vi "Configure TLS.vi"(4 "Cert Chain Format":enum32{"X.509 (PEM)"}(ring), 6 "Cert Chain Path":path, 7 "Private Key Password":string, 8 "error in (no error)":errorcluster, 9 "Private Key Format":enum32{"PKCS#8 (PEM)", "PKCS#8 (DER)"}(ring), 10 "Private Key Path":path, 11 "Websocket Server in":refnum<class "Websocket Server.lvclass">) -> (0 "error out":errorcluster, 3 "Websocket Server out":refnum<class "Websocket Server.lvclass">)   [LabVIEW 2020, in "Stream-Websocket.lvlib" / "Websocket Server.lvclass"]
uses:
  Websocket Server.lvclass
  Websocket Server.lvclass/Websocket Server.ctl
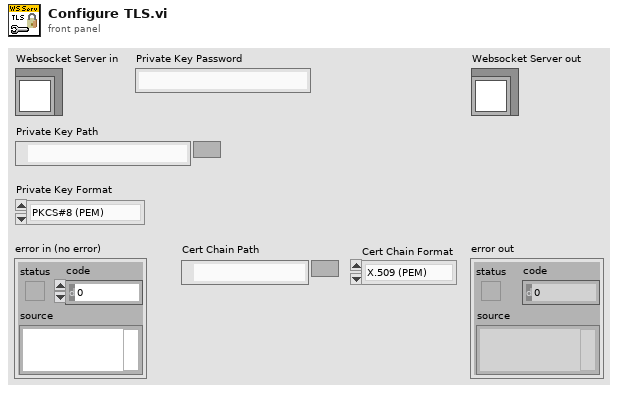
[diagram p1: front panel]
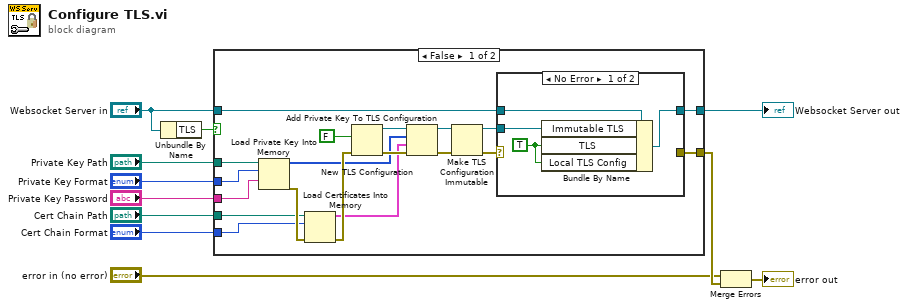
[diagram p0: block diagram]
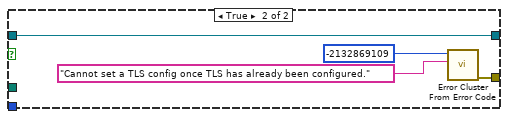
[diagram p3: hidden frame]
diagram:
  n1 = Unbundle By Name("Websocket Server in") -> ("TLS"=w3:bool)
  n2 = case shown="False" w3 {
    tunnel: "Cert Chain Path" -> [w29 _]
    tunnel: "Cert Chain Format" -> [w28 _]
    tunnel: "Private Key Format" -> [w27 _]
    tunnel: "Private Key Path" -> [w26 _]
    tunnel: "Private Key Password" -> [w25 _]
    tunnel: "Websocket Server in" -> [w14 w40]
    tunnel: [w12 w40] -> w4
    tunnel: [w15 w37] -> w6
    frame False {
      n3 = Load Private Key Into Memory(9:w25, 10:w27, 11:w26) -> (0:w30:errorcluster, 3:w20:u8[])  [unwired: 1 in]
      n4 = Load Certificates Into Memory(8:w30, 10:w28, 11:w29) -> (0:w23:errorcluster, 3:w19:cluster{"certificate":u8[]}[])
      n5 = New TLS Configuration(8:w23, 10:FALSE ("load OS trusted CAs?")) -> (0:w22:errorcluster, 3:w21:refnum<k36>)
      n6 = Add Private Key To TLS Configuration(8:w22, 9:w19, 10:w20, 11:w21) -> (0:w18:errorcluster, 3:w17:refnum<k36>)
      n7 = Make TLS Configuration Immutable(8:w18, 11:w17) -> (0:w16:errorcluster, 3:w13:refnum<k36>)
      n8 = case shown="No Error" w16 {
        selector: w16 -> [_ w36]
        tunnel: [_ w36] -> w15
        tunnel: w14 -> [w34 w35]
        tunnel: w13 -> [w33 _]
        tunnel: [w32 w35] -> w12
        frame No Error {
          w31 = TRUE ("TLS")
          n9 = Bundle By Name(cluster=w34, "Immutable TLS"=w33, "TLS"=w31, "Local TLS Config"=w31) -> (w32:refnum<class "Websocket Server.lvclass">)
        }
        frame Error {
        }
      }
    }
    frame True {
      n10 = call <vilib>:"Error Cluster From Error Code.vi"("error message (\"\")"="Cannot set a TLS config once TLS has already been configured." ("error message (\"\")"), "error code (0)"=-2132869109) -> ("error out"=w37:errorcluster)  [unwired: 7 in]
    }
  }
  "Websocket Server out" <- w4
  n11 = Merge Errors("error in (no error)", w6) -> (→"error out":errorcluster)
